vi "ValidateStringInFile.vi"(9 "Data Column (0)":dbl, 10 "String to find":string, 11 "Path In":path) -> (1 "Data File Found":bool, 2 "String Found":bool, 3 "String Out":string)   [LabVIEW 2024, in "LVarex.lvlib"]
uses:
  <vilib>/Utility/error.llb/Trim Whitespace One-Sided.vi
  <vilib>/Utility/file.llb/Read Delimited Spreadsheet (string).vi
  LVarex.lvlib
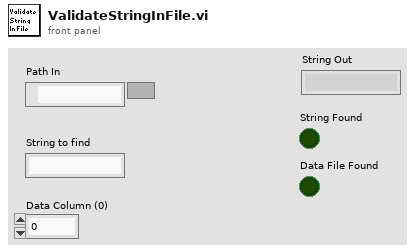
[diagram p1: front panel]
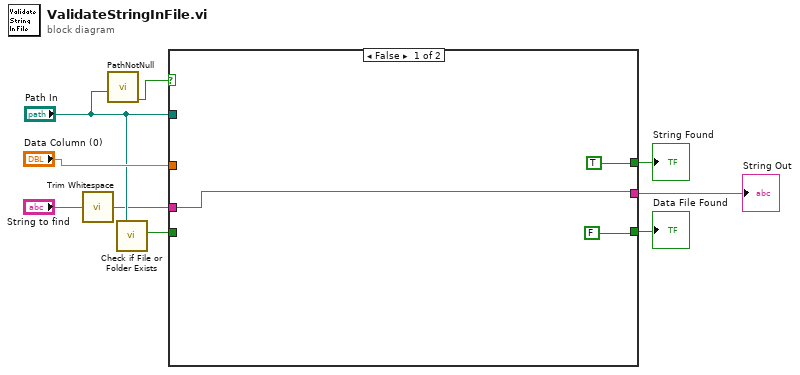
[diagram p0: block diagram]
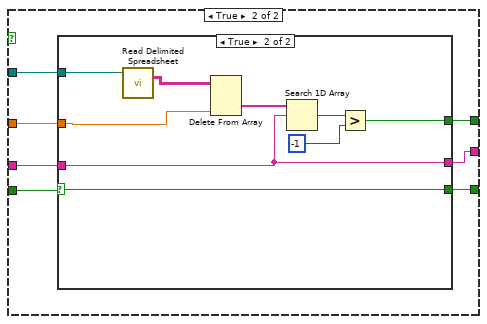
[diagram p2: hidden frame]
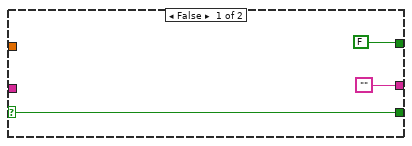
[diagram p3: hidden frame]
diagram:
  n1 = call <vilib>:"Trim Whitespace.vi"("string"="String to find") -> ("trimmed string"=w1:string)  [unwired: 1 in]
  n2 = call "PathNotNull.vi"("Path In"="Path In") -> ("Not Null Out"=w3:bool)  [unwired: 10 in]
  n3 = call <vilib>:"Check if File or Folder Exists.vi"("path"="Path In") -> ("file or folder exists?"=w9:bool)  [unwired: 8 in, 2 out]
  n4 = case shown="False" w3 {
    tunnel: "Path In" -> [_ w19]
    tunnel: w9 -> [_ w18]
    tunnel: "Data Column (0)" -> [_ w17]
    tunnel: w1 -> [w10 w16]
    tunnel: [TRUE w15] -> w7
    tunnel: [FALSE w14] -> w6
    tunnel: [w10 w13] -> w5
    frame False {
    }
    frame True {
      n5 = case shown="True" w18 {
        selector: w18 -> [w22 w24]
        tunnel: w19 -> [_ w31]
        tunnel: w17 -> [_ w29]
        tunnel: w16 -> [_ w23]
        tunnel: [FALSE w25] -> w15
        tunnel: [w22 w24] -> w14
        tunnel: ["" w23] -> w13
        frame False {
        }
        frame True {
          n6 = call-poly <vilib>:"Read Delimited Spreadsheet.vi"("file path (dialog if empty)"=w31) -> ("all rows"=w30:string[][])  [unwired: 9 in, 5 out]
          n7 = Delete From Array(array=w30, index (col)=w29) -> (deleted portion=w28:string[])  [unwired: 2 in, 1 out]
          n8 = Search 1D Array(1D array=w28, element=w23) -> (index of element=w27:i32)  [unwired: 1 in]
          n9 = Greater?(x=w27, y=-1) -> (0:w25:bool)
        }
      }
    }
  }
  "String Out" <- w5
  "String Found" <- w7
  "Data File Found" <- w6
